vi "AMWave.vi"() -> ()   [LabVIEW 2015]
panel:
  in  "Amplitude":dbl
  in  "Modulation Frequency":dbl
  in  "Signal Frequency":dbl
  in  "Sampling Frequency":dbl
  in  "Number of Samples":dbl
  out "XY Graph":cluster{"t":dbl[], "x":dbl[]}(graph)
  # "Digitizing Parameters"
  # "AM Wave"
  # "AM Wave Parameters"
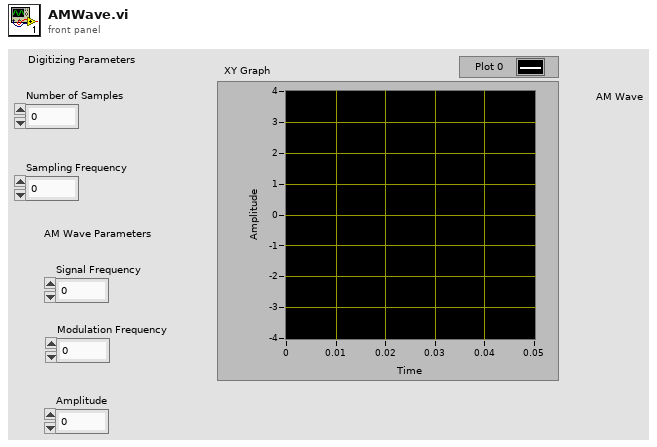
[diagram p1: front panel]
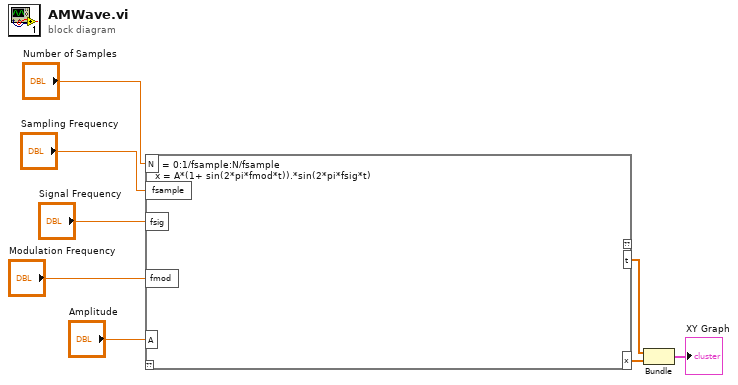
[diagram p0: block diagram]
diagram:
  n1 = mathscript code="t = 0:1/fsample:N/fsample\nx = A*(1+ sin(2*pi*fmod*t)).*sin(2*pi*fsig*t)"("fmod"="Modulation Frequency", "fsig"="Signal Frequency", "N"="Number of Samples", "A"="Amplitude", "fsample"="Sampling Frequency") -> ("t"=w3:dbl[], "x"=w2:dbl[])  [unwired: 1 in, 1 out]
  n2 = Bundle("t"=w3, "x"=w2) -> (→"XY Graph":cluster{"t":dbl[], "x":dbl[]})  [unwired: 1 in]
